vi "VISetDirectionDigital.vi"(1 "Enable Digital Output":u32, 2 "FPGA Interface Input":refnum<k20>) -> ()   [LabVIEW 2012]
uses:
  <vilib>/Utility/error.llb/Error Cluster From Error Code.vi
  <vilib>/rvi/errors/niLvFpgaAdjustHostInterfaceError.vi
  <vilib>/rvi/interface/nirviReadWriteControl/nirviReadWriteControl.xnode
  NiFpgaLv.dll
  <vilib>/rvi/interface/Simulation/niFpgaSimulationCallBeginRW.vi
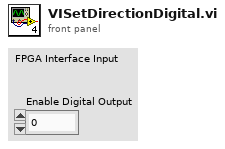
[diagram p1: front panel]
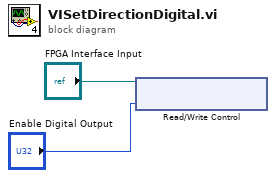
[diagram p0: block diagram]
diagram:
  n1 = xnode "Read/Write Control"("FPGA VI Reference In"="FPGA Interface Input", "Enable Digital Output"="Enable Digital Output") -> ()  [unwired: 1 in, 2 out]
